vi "closeAVI.vi"(8 "error in (no error)":errorcluster, 11 "Input cluster":T1) -> (0 "error out":errorcluster, 3 "Output cluster":T1)   [LabVIEW 2020]
uses:
  controls/StateMachineVariables.ctl
  <vilib>/vision/Avi.llb/IMAQ AVI2 Refnum.ctl
  <vilib>/userDefined/High Color/IMAQdx.ctl
  <vilib>/vision/Deep Learning.llb/IMAQ DL Model Refnum.ctl
  <vilib>/vision/Image Controls.llb/IMAQ Image.ctl
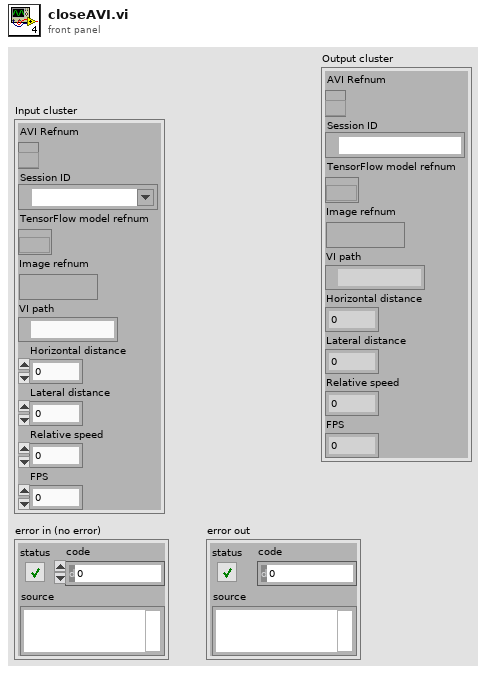
[diagram p1: front panel]
types:
  T1 = typedef "StateMachineVariables.ctl" = cluster{"AVI Refnum":T2, "Session ID":T3, "TensorFlow model refnum":T4, "Image refnum":T5, "VI path":path, "Horizontal distance":dbl, "Lateral distance":dbl, "Relative speed":dbl, "FPS":dbl}
  T2 = typedef "IMAQ AVI2 Refnum.ctl" = refnum<k20>
  T3 = typedef "IMAQdx.ctl" = refnum<k21>
  T4 = typedef "IMAQ DL Model Refnum.ctl" = refnum<k20>
  T5 = typedef "IMAQ Image.ctl" = refnum<image>
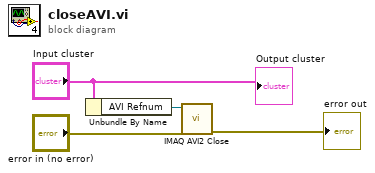
[diagram p0: block diagram]
diagram:
  n1 = Unbundle By Name("Input cluster") -> ("AVI Refnum"=w4:T2)
  n2 = call "IMAQ AVI2 Close"("error in (no error)"="error in (no error)", "AVI Refnum"=w4) -> ("error out"=→"error out":errorcluster)  [unwired: 9 in]
  "Output cluster" <- "Input cluster"
